vi "Update Tag Integer.vi"(8 "error in (no error)":errorcluster, 9 "Value":i32, 10 "Tag Path":string, 11 "Logger in.lvclass":refnum<class "Logger.lvclass">) -> (0 "error out":errorcluster, 3 "Logger out.lvclass":refnum<class "Logger.lvclass">)   [LabVIEW 2021, in "Logger.lvclass"]
uses:
  Logger.lvclass
  Logger.lvclass/Logger.ctl
  <vilib>/Skyline/Tag/Wrapper/Wrapper_class/Generate Tag Cluster (I32) 2.vi
  <vilib>/Waveform/WDTOps.llb/Number of Waveform Samples.vi
  <vilib>/Waveform/WDTOps.llb/WDT Number of Waveform Samples DBL.vi
  <vilib>/Skyline/Tag/Wrapper/Wrapper_class/Generate Tag Cluster Core 2.vi
  <vilib>/Skyline/Tag/Wrapper/Wrapper_class/NI Skyline Tag.lvclass
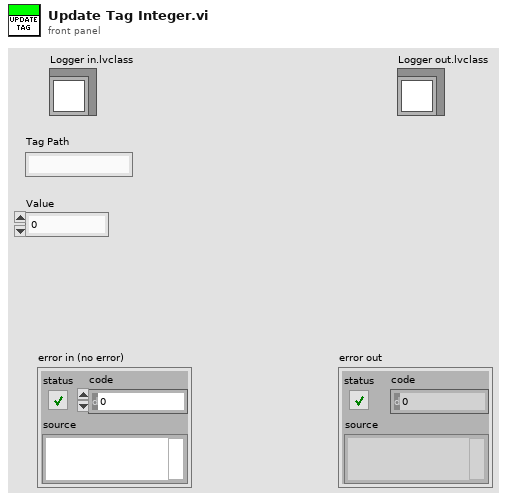
[diagram p1: front panel]
types:
  T1 = cluster{"Tag Units":string, "Tag Path":string, "Waveform":waveform(dbl), "Log":bool, "Tag Reference":refnum<class "NI Skyline Tag.lvclass">}[]
  T2 = typedef "NI Skyline Tag.lvclass/Tag Value Cluster Wrapper.ctl" = cluster{"Configuration":refnum<class "NI Skyline Configuration.lvclass">, "Tag Cluster":T3}
  T3 = typedef "NI Skyline Tag.lvlib/Tag Value Cluster.ctl" = cluster{"Path":string, "Workspace ID":string, "Data Type":T4, "Value":string, "Time Stamp":timestamp}
  T4 = typedef "NI Skyline Tag.lvlib/DataType.ctl" = enum32{"Double", "I32", "String", "Boolean", "U64", "Timestamp"}
  T5 = cluster{"Tag Units":string, "Tag Path":string, "Waveform":waveform(dbl), "Log":bool, "Tag Reference":refnum<class "NI Skyline Tag.lvclass">}
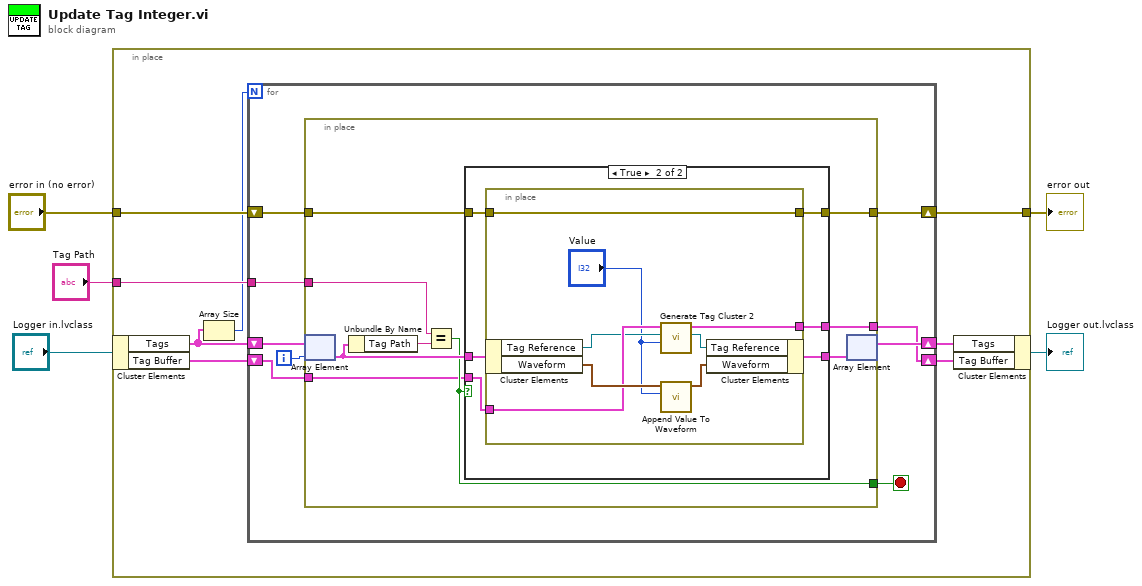
[diagram p0: block diagram]
diagram:
  n1 = in-place {
    in-place-border: "Tag Path" -> [w13]
    in-place-border: "error in (no error)" -> [w11]
    in-place-border: [w10] -> w1
    n2 = in-place-cluster #1("Logger in.lvclass") -> ("Tags"=w6:T1, "Tag Buffer"=w8:T2[])
    n3 = Array Size(array=w6) -> (size(s)=w9:i32)
    n4 = for {
      N: w9 -> [_]
      tunnel: w13 -> [w22]
      shift-right: [w19] -> w12
      shift-left: w6 -> [w21]
      shift-right: [w17] -> w10
      shift-left: w11 -> [w18]
      shift-right: [w14] -> w7
      shift-left: w8 -> [w15]
      i -> [w20]
      stop <- w16 stop-if-true
      n5 = in-place {
        in-place-border: w22 -> [w27]
        in-place-border: [w25] -> w16
        in-place-border: w18 -> [w29]
        in-place-border: [w28] -> w17
        in-place-border: w15 -> [w24]
        in-place-border: [w23] -> w14
        n6 = in-place-array #2(w21, w20) -> (w30:T5)
        n7 = Unbundle By Name(w30) -> ("Tag Path"=w26:string)
        n8 = Equal?(x=w27, y=w26) -> (x = y?=w25:bool)
        n9 = case shown="True" w25 {
          tunnel: w30 -> [w34 w40]
          tunnel: [w34 w39] -> w31
          tunnel: w29 -> [w33 w38]
          tunnel: [w33 w36] -> w28
          tunnel: w24 -> [w32 w37]
          tunnel: [w32 w35] -> w23
          frame False {
          }
          frame True {
            n10 = in-place {
              in-place-border: w38 -> [w46]
              in-place-border: w37 -> [w45]
              in-place-border: [w46] -> w36
              in-place-border: [w44] -> w35
              n11 = in-place-cluster #3(w40) -> ("Tag Reference"=w43:refnum<class "NI Skyline Tag.lvclass">, "Waveform"=w48:waveform(dbl))
              n12 = call-poly <vilib>:"Generate Tag Cluster 2.vi"("value"="Value", "tag in"=w43, "tag clusters in"=w45) -> ("tag out"=w41:refnum<class "NI Skyline Tag.lvclass">, "tag clusters out"=w44:T2[])  [unwired: 6 in, 1 out]
              n13 = call "Append Value To Waveform.vi"("Numeric"="Value", "waveform in"=w48) -> ("waveform out"=w47:waveform(dbl))  [unwired: 9 in]
              n14 = in-place-cluster #3("Tag Reference"=w41, "Waveform"=w47) -> (w39:T5)
            }
          }
        }
        n15 = in-place-array #2(w31) -> (w19:T1)  [unwired: 1 out]
      }
    }
    n16 = in-place-cluster #1("Tags"=w12, "Tag Buffer"=w7) -> (→"Logger out.lvclass":refnum<class "Logger.lvclass">)
  }
  "error out" <- w1
